vi "Camera device types.vi"() -> (3 "Camera device types":string[](array[string]))   [LabVIEW 2020]
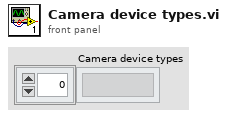
[diagram p1: front panel]
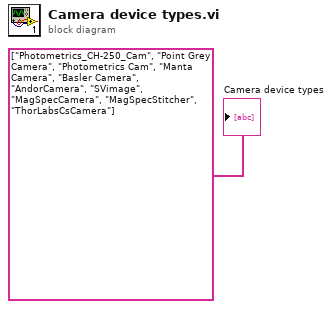
[diagram p0: block diagram]
diagram:
  "Camera device types" <- string[] ["Photometrics_CH-250_Cam", "Point Grey Camera", "Photometrics Cam", "Manta Camera", "Basler Camera", "AndorCamera", "SVimage", "MagSpecCamera", "MagSpecStitcher", "ThorLabsCsCamera"]
